vi "Message Packet To Class.vi"(8 "error in":errorcluster, 11 "Message Packet":T1) -> (0 "error out":errorcluster, 2 "Error?":bool, 3 "SECS-II Class":refnum<class "SECS-II Class.lvclass">)   [LabVIEW 2020, in "SECS Communication.lvlib" / "HSMS Class.lvclass"]
uses:
  HSMS Class.lvclass
  Message Packet.ctl
  SECS-II Class/SECS-II Class.lvclass
  SECS-II Class/SECS-II Class.lvclass/SECS-II Class.ctl
  S1 Message Class/S1 Message Class.lvclass
  D:/Dropbox/SECS/SECS_GEM v1.1.0/Com/SECS Communication/SECS-II Class/SECS-II Class.lvclass
  S2 Message Class/S2 Message Class.lvclass
  S3 Message Class/S3 Message Class.lvclass
  S4 Message Class/S4 Message Class.lvclass
  S5 Message Class/S5 Message Class.lvclass
  S6 Message Class/S6 Message Class.lvclass
  S7 Message Class/S7 Message Class.lvclass
  S8 Message Class/S8 Message Class.lvclass
  S9 Message Class/S9 Message Class.lvclass
  S10 Message Class/S10 Message Class.lvclass
  SECS-II Class/Write System Btyes.vi
  SECS-II Class/Write Message Header.vi
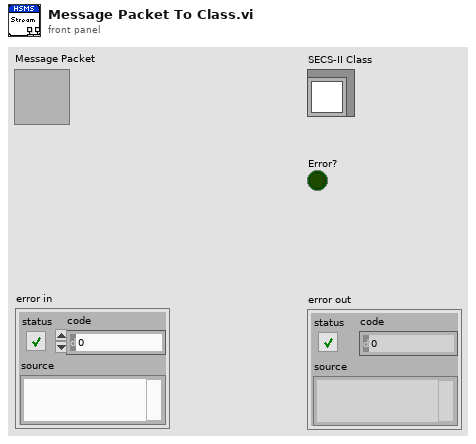
[diagram p1: front panel]
types:
  T1 = typedef "SECS Communication.lvlib/HSMS Class.lvclass/Message Packet.ctl" = cluster{"Message Header Cluster":T2, "Message Header":u8[], "Message Text":u8[]}
  T2 = typedef "SECS Communication.lvlib/HSMS Class.lvclass/Message Header.ctl" = cluster{"Byte 0-1(Session ID)":u16, "W-Bit":bool, "Byte 2":u8, "Byte 3":u8, "Byte 4(PType)":T3, "Byte 5(SType)":T4, "Byte 6-9(System Btyes)":u8[]}
  T3 = typedef "SECS Communication.lvlib/HSMS Class.lvclass/PType.ctl" = enum8{"SECS-II Encoding", "Reserved"}
  T4 = typedef "SECS Communication.lvlib/HSMS Class.lvclass/SType.ctl" = enum8{"Data Message", "Select.req", "Select.rsp", "Deselect.req", "Deselect.rsp", "Linktest.req", "Linktest.rsp", "Reject.req", "Separate.req"}
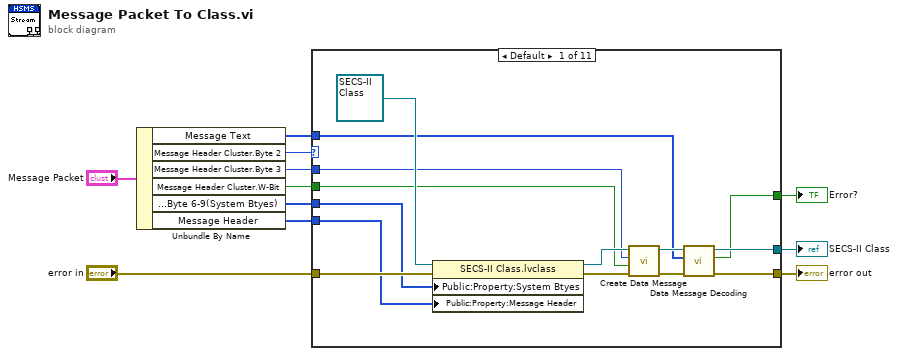
[diagram p0: block diagram]
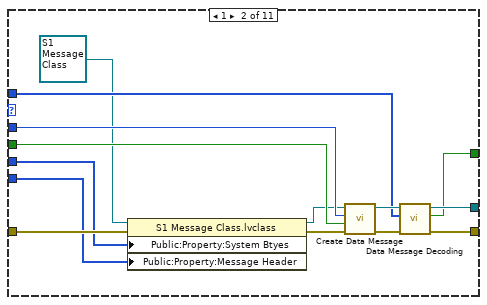
[diagram p2: hidden frame]
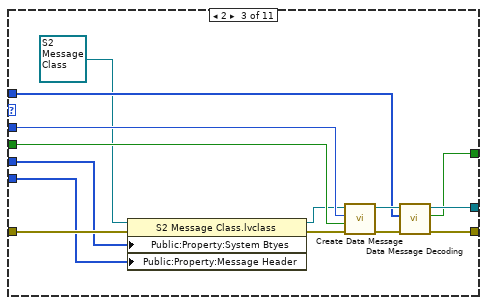
[diagram p3: hidden frame]
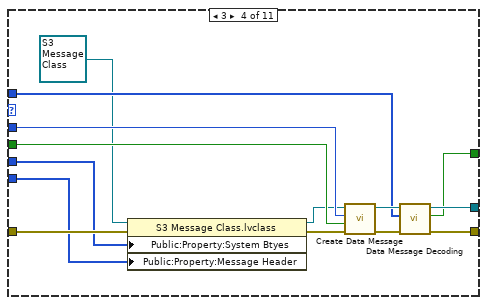
[diagram p4: hidden frame]
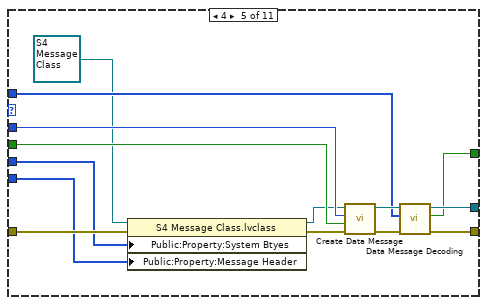
[diagram p5: hidden frame]
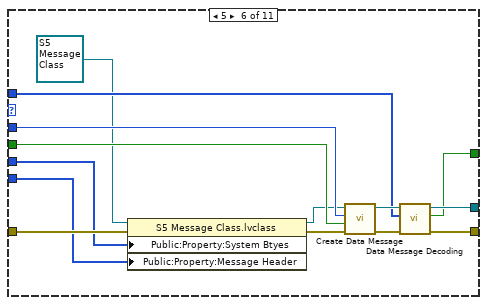
[diagram p6: hidden frame]
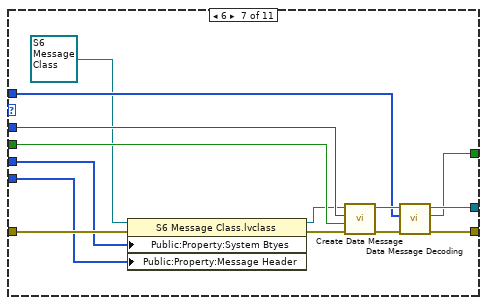
[diagram p7: hidden frame]
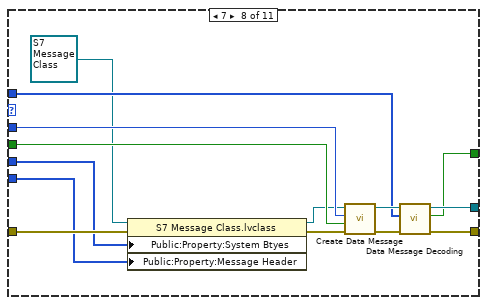
[diagram p8: hidden frame]
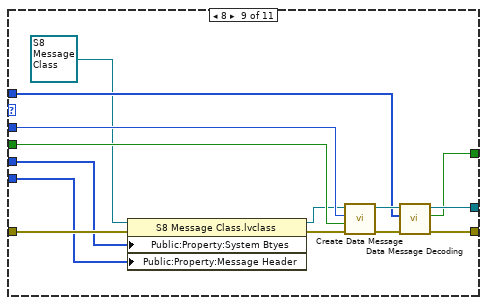
[diagram p9: hidden frame]
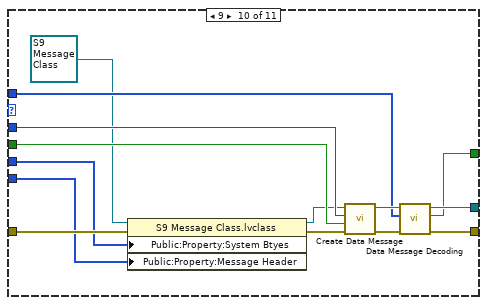
[diagram p10: hidden frame]
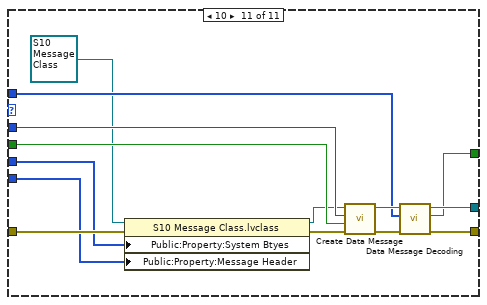
[diagram p11: hidden frame]
diagram:
  n1 = Unbundle By Name("Message Packet") -> ("Message Text"=w8:u8[], "Message Header Cluster.Byte 2"=w3:u8, "Message Header Cluster.Byte 3"=w9:u8, "Message Header Cluster.W-Bit"=w10:bool, "Message Header Cluster.Byte 6-9(System Btyes)"=w2:u8[], "Message Header"=w1:u8[])
  n2 = case shown="Default" w3 {
    tunnel: "error in" -> [w21 w31 w45 w59 w73 w87 w101 w115 w129 w143 w157]
    tunnel: w10 -> [w18 w39 w53 w67 w81 w95 w109 w123 w137 w151 w165]
    tunnel: w9 -> [w19 w38 w52 w66 w80 w94 w108 w122 w136 w150 w164]
    tunnel: w8 -> [w16 w35 w49 w63 w77 w91 w105 w119 w133 w147 w161]
    tunnel: [w14 w34 w48 w62 w76 w90 w104 w118 w132 w146 w160] -> w6
    tunnel: [w17 w33 w47 w61 w75 w89 w103 w117 w131 w145 w159] -> w5
    tunnel: [w15 w32 w46 w60 w74 w88 w102 w116 w130 w144 w158] -> w4
    tunnel: w2 -> [w13 w27 w41 w55 w70 w84 w98 w112 w126 w140 w154]
    tunnel: w1 -> [w12 w26 w40 w54 w68 w82 w96 w110 w124 w138 w152]
    frame Default {
      n3 = property class="SECS-II Class.lvclass"(reference=refnum<class "SECS-II Class.lvclass"> refnum ("SECS Communication.lvlib:SECS-II Class.lvclass"), error in=w21, "Public:Property:System Btyes"=w13, "Public:Property:Message Header"=w12) -> (reference out=w22:refnum<class "SECS-II Class.lvclass">, error out=w23:errorcluster)
      n4 = call "Create Data Message.vi"("error in (no error)"=w23, "W-Bit"=w18, "Function"=w19, "SECS-II Class in"=w22) -> ("error out"=w25:errorcluster, "SECS-II Class out"=w24:refnum<class "SECS-II Class.lvclass">)  [unwired: 6 in]
      n5 = call "Data Message Decoding.vi"("error in"=w25, "Message Text"=w16, "SECS-II Class in"=w24) -> ("error out"=w14:errorcluster, "Error?"=w15:bool, "SECS-II Class out"=w17:refnum<class "SECS-II Class.lvclass">)  [unwired: 6 in]
    }
    frame 1 {
      n6 = property class="S1 Message Class.lvclass"(reference=refnum<class "S1 Message Class.lvclass"> refnum ("SECS Communication.lvlib:S1 Message Class.lvclass"), error in=w31, "Public:Property:System Btyes"=w27, "Public:Property:Message Header"=w26) -> (reference out=w28:refnum<class "S1 Message Class.lvclass">, error out=w29:errorcluster)
      n7 = call "Create Data Message.vi"("error in (no error)"=w29, "W-Bit"=w39, "Function"=w38, "SECS-II Class in"=w28) -> ("error out"=w37:errorcluster, "SECS-II Class out"=w36:refnum<class "S1 Message Class.lvclass">)  [unwired: 6 in]
      n8 = call "Data Message Decoding.vi"("error in"=w37, "Message Text"=w35, "SECS-II Class in"=w36) -> ("error out"=w34:errorcluster, "Error?"=w32:bool, "SECS-II Class out"=w33:refnum<class "S1 Message Class.lvclass">)  [unwired: 6 in]
    }
    frame 2 {
      n9 = property class="S2 Message Class.lvclass"(reference=refnum<class "S2 Message Class.lvclass"> refnum ("SECS Communication.lvlib:S2 Message Class.lvclass"), error in=w45, "Public:Property:System Btyes"=w41, "Public:Property:Message Header"=w40) -> (reference out=w42:refnum<class "S2 Message Class.lvclass">, error out=w43:errorcluster)
      n10 = call "Create Data Message.vi"("error in (no error)"=w43, "W-Bit"=w53, "Function"=w52, "SECS-II Class in"=w42) -> ("error out"=w51:errorcluster, "SECS-II Class out"=w50:refnum<class "S2 Message Class.lvclass">)  [unwired: 6 in]
      n11 = call "Data Message Decoding.vi"("error in"=w51, "Message Text"=w49, "SECS-II Class in"=w50) -> ("error out"=w48:errorcluster, "Error?"=w46:bool, "SECS-II Class out"=w47:refnum<class "S2 Message Class.lvclass">)  [unwired: 6 in]
    }
    frame 3 {
      n12 = property class="S3 Message Class.lvclass"(reference=refnum<class "S3 Message Class.lvclass"> refnum ("SECS Communication.lvlib:S3 Message Class.lvclass"), error in=w59, "Public:Property:System Btyes"=w55, "Public:Property:Message Header"=w54) -> (reference out=w56:refnum<class "S3 Message Class.lvclass">, error out=w57:errorcluster)
      n13 = call "Create Data Message.vi"("error in (no error)"=w57, "W-Bit"=w67, "Function"=w66, "SECS-II Class in"=w56) -> ("error out"=w65:errorcluster, "SECS-II Class out"=w64:refnum<class "S3 Message Class.lvclass">)  [unwired: 6 in]
      n14 = call "Data Message Decoding.vi"("error in"=w65, "Message Text"=w63, "SECS-II Class in"=w64) -> ("error out"=w62:errorcluster, "Error?"=w60:bool, "SECS-II Class out"=w61:refnum<class "S3 Message Class.lvclass">)  [unwired: 6 in]
    }
    frame 4 {
      n15 = property class="S4 Message Class.lvclass"(reference=refnum<class "S4 Message Class.lvclass"> refnum ("SECS Communication.lvlib:S4 Message Class.lvclass"), error in=w73, "Public:Property:System Btyes"=w70, "Public:Property:Message Header"=w68) -> (reference out=w71:refnum<class "S4 Message Class.lvclass">, error out=w72:errorcluster)
      n16 = call "Create Data Message.vi"("error in (no error)"=w72, "W-Bit"=w81, "Function"=w80, "SECS-II Class in"=w71) -> ("error out"=w79:errorcluster, "SECS-II Class out"=w78:refnum<class "S4 Message Class.lvclass">)  [unwired: 6 in]
      n17 = call "Data Message Decoding.vi"("error in"=w79, "Message Text"=w77, "SECS-II Class in"=w78) -> ("error out"=w76:errorcluster, "Error?"=w74:bool, "SECS-II Class out"=w75:refnum<class "S4 Message Class.lvclass">)  [unwired: 6 in]
    }
    frame 5 {
      n18 = property class="S5 Message Class.lvclass"(reference=refnum<class "S5 Message Class.lvclass"> refnum ("SECS Communication.lvlib:S5 Message Class.lvclass"), error in=w87, "Public:Property:System Btyes"=w84, "Public:Property:Message Header"=w82) -> (reference out=w85:refnum<class "S5 Message Class.lvclass">, error out=w86:errorcluster)
      n19 = call "Create Data Message.vi"("error in (no error)"=w86, "W-Bit"=w95, "Function"=w94, "SECS-II Class in"=w85) -> ("error out"=w93:errorcluster, "SECS-II Class out"=w92:refnum<class "S5 Message Class.lvclass">)  [unwired: 6 in]
      n20 = call "Data Message Decoding.vi"("error in"=w93, "Message Text"=w91, "SECS-II Class in"=w92) -> ("error out"=w90:errorcluster, "Error?"=w88:bool, "SECS-II Class out"=w89:refnum<class "S5 Message Class.lvclass">)  [unwired: 6 in]
    }
    frame 6 {
      n21 = property class="S6 Message Class.lvclass"(reference=refnum<class "S6 Message Class.lvclass"> refnum ("SECS Communication.lvlib:S6 Message Class.lvclass"), error in=w101, "Public:Property:System Btyes"=w98, "Public:Property:Message Header"=w96) -> (reference out=w99:refnum<class "S6 Message Class.lvclass">, error out=w100:errorcluster)
      n22 = call "Create Data Message.vi"("error in (no error)"=w100, "W-Bit"=w109, "Function"=w108, "SECS-II Class in"=w99) -> ("error out"=w107:errorcluster, "SECS-II Class out"=w106:refnum<class "S6 Message Class.lvclass">)  [unwired: 6 in]
      n23 = call "Data Message Decoding.vi"("error in"=w107, "Message Text"=w105, "SECS-II Class in"=w106) -> ("error out"=w104:errorcluster, "Error?"=w102:bool, "SECS-II Class out"=w103:refnum<class "S6 Message Class.lvclass">)  [unwired: 6 in]
    }
    frame 7 {
      n24 = property class="S7 Message Class.lvclass"(reference=refnum<class "S7 Message Class.lvclass"> refnum ("SECS Communication.lvlib:S7 Message Class.lvclass"), error in=w115, "Public:Property:System Btyes"=w112, "Public:Property:Message Header"=w110) -> (reference out=w113:refnum<class "S7 Message Class.lvclass">, error out=w114:errorcluster)
      n25 = call "Create Data Message.vi"("error in (no error)"=w114, "W-Bit"=w123, "Function"=w122, "SECS-II Class in"=w113) -> ("error out"=w121:errorcluster, "SECS-II Class out"=w120:refnum<class "S7 Message Class.lvclass">)  [unwired: 6 in]
      n26 = call "Data Message Decoding.vi"("error in"=w121, "Message Text"=w119, "SECS-II Class in"=w120) -> ("error out"=w118:errorcluster, "Error?"=w116:bool, "SECS-II Class out"=w117:refnum<class "S7 Message Class.lvclass">)  [unwired: 6 in]
    }
    frame 8 {
      n27 = property class="S8 Message Class.lvclass"(reference=refnum<class "S8 Message Class.lvclass"> refnum ("SECS Communication.lvlib:S8 Message Class.lvclass"), error in=w129, "Public:Property:System Btyes"=w126, "Public:Property:Message Header"=w124) -> (reference out=w127:refnum<class "S8 Message Class.lvclass">, error out=w128:errorcluster)
      n28 = call "Create Data Message.vi"("error in (no error)"=w128, "W-Bit"=w137, "Function"=w136, "SECS-II Class in"=w127) -> ("error out"=w135:errorcluster, "SECS-II Class out"=w134:refnum<class "S8 Message Class.lvclass">)  [unwired: 6 in]
      n29 = call "Data Message Decoding.vi"("error in"=w135, "Message Text"=w133, "SECS-II Class in"=w134) -> ("error out"=w132:errorcluster, "Error?"=w130:bool, "SECS-II Class out"=w131:refnum<class "S8 Message Class.lvclass">)  [unwired: 6 in]
    }
    frame 9 {
      n30 = property class="S9 Message Class.lvclass"(reference=refnum<class "S9 Message Class.lvclass"> refnum ("SECS Communication.lvlib:S9 Message Class.lvclass"), error in=w143, "Public:Property:System Btyes"=w140, "Public:Property:Message Header"=w138) -> (reference out=w141:refnum<class "S9 Message Class.lvclass">, error out=w142:errorcluster)
      n31 = call "Create Data Message.vi"("error in (no error)"=w142, "W-Bit"=w151, "Function"=w150, "SECS-II Class in"=w141) -> ("error out"=w149:errorcluster, "SECS-II Class out"=w148:refnum<class "S9 Message Class.lvclass">)  [unwired: 6 in]
      n32 = call "Data Message Decoding.vi"("error in"=w149, "Message Text"=w147, "SECS-II Class in"=w148) -> ("error out"=w146:errorcluster, "Error?"=w144:bool, "SECS-II Class out"=w145:refnum<class "S9 Message Class.lvclass">)  [unwired: 6 in]
    }
    frame 10 {
      n33 = property class="S10 Message Class.lvclass"(reference=refnum<class "S10 Message Class.lvclass"> refnum ("SECS Communication.lvlib:S10 Message Class.lvclass"), error in=w157, "Public:Property:System Btyes"=w154, "Public:Property:Message Header"=w152) -> (reference out=w155:refnum<class "S10 Message Class.lvclass">, error out=w156:errorcluster)
      n34 = call "Create Data Message.vi"("error in (no error)"=w156, "W-Bit"=w165, "Function"=w164, "SECS-II Class in"=w155) -> ("error out"=w163:errorcluster, "SECS-II Class out"=w162:refnum<class "S10 Message Class.lvclass">)  [unwired: 6 in]
      n35 = call "Data Message Decoding.vi"("error in"=w163, "Message Text"=w161, "SECS-II Class in"=w162) -> ("error out"=w160:errorcluster, "Error?"=w158:bool, "SECS-II Class out"=w159:refnum<class "S10 Message Class.lvclass">)  [unwired: 6 in]
    }
  }
  "error out" <- w6
  "SECS-II Class" <- w5
  "Error?" <- w4
